vi "CRYImp wiz p2 basic format.vi"(5 "Iteration":i32, 6 "x-y settings array":T1 {"yp db ref" format="%.2f"; "ym db ref" format="%.2f"; "x db ref" format="%.2f"}, 7 "Flat data in (optional)":string, 8 "error in (no error)":errorcluster, 10 "Main info cluster":T2, 11 "Page flags":T3) -> (0 "error out":errorcluster, 1 "Data out":string[][](array[string]), 2 "Main info cluster out":T2, 3 "Page flags out":T3, 4 "x-y settings array out":T1 {"yp db ref" format="%.2f"; "ym db ref" format="%.2f"; "x db ref" format="%.2f"})   [LabVIEW 2013]
uses:
  Control/CRYImp wiz page flags.ctl
  Control/CRYImp wiz main info.ctl
  Control/CRYx-y settings array.ctl
panel:
  out "Operand_A1":bool
  in  "column width:":i32=10 caption="列宽度:"
  in  "col oth delim":string="   " caption="其他:"
  in  "column delimiter:":u16(ring) caption="aa" items=["tab", "comma", "space", "other"]
  in  "prev":bool
  in  "next":bool
  in  "cancel":bool
  in  "finish":bool
  in  "rows/cols":i32(slide) caption="aa"
  in  "file format":i32(slide)
  in  "offset cols":i32 caption="aa" min=0
  in  "offset rows":i32 caption="aa" min=0
  out "File viewer (after offset):":string[][](table) caption="aa"
  in  "cont":bool
  in  "header col":i32=1 caption="行/列:" min=1
  in  "header":bool caption="aaa"
  in  "load":bool
  in  "cntls update":bool
  in  "std hdr":bool caption="标准头包含轴"
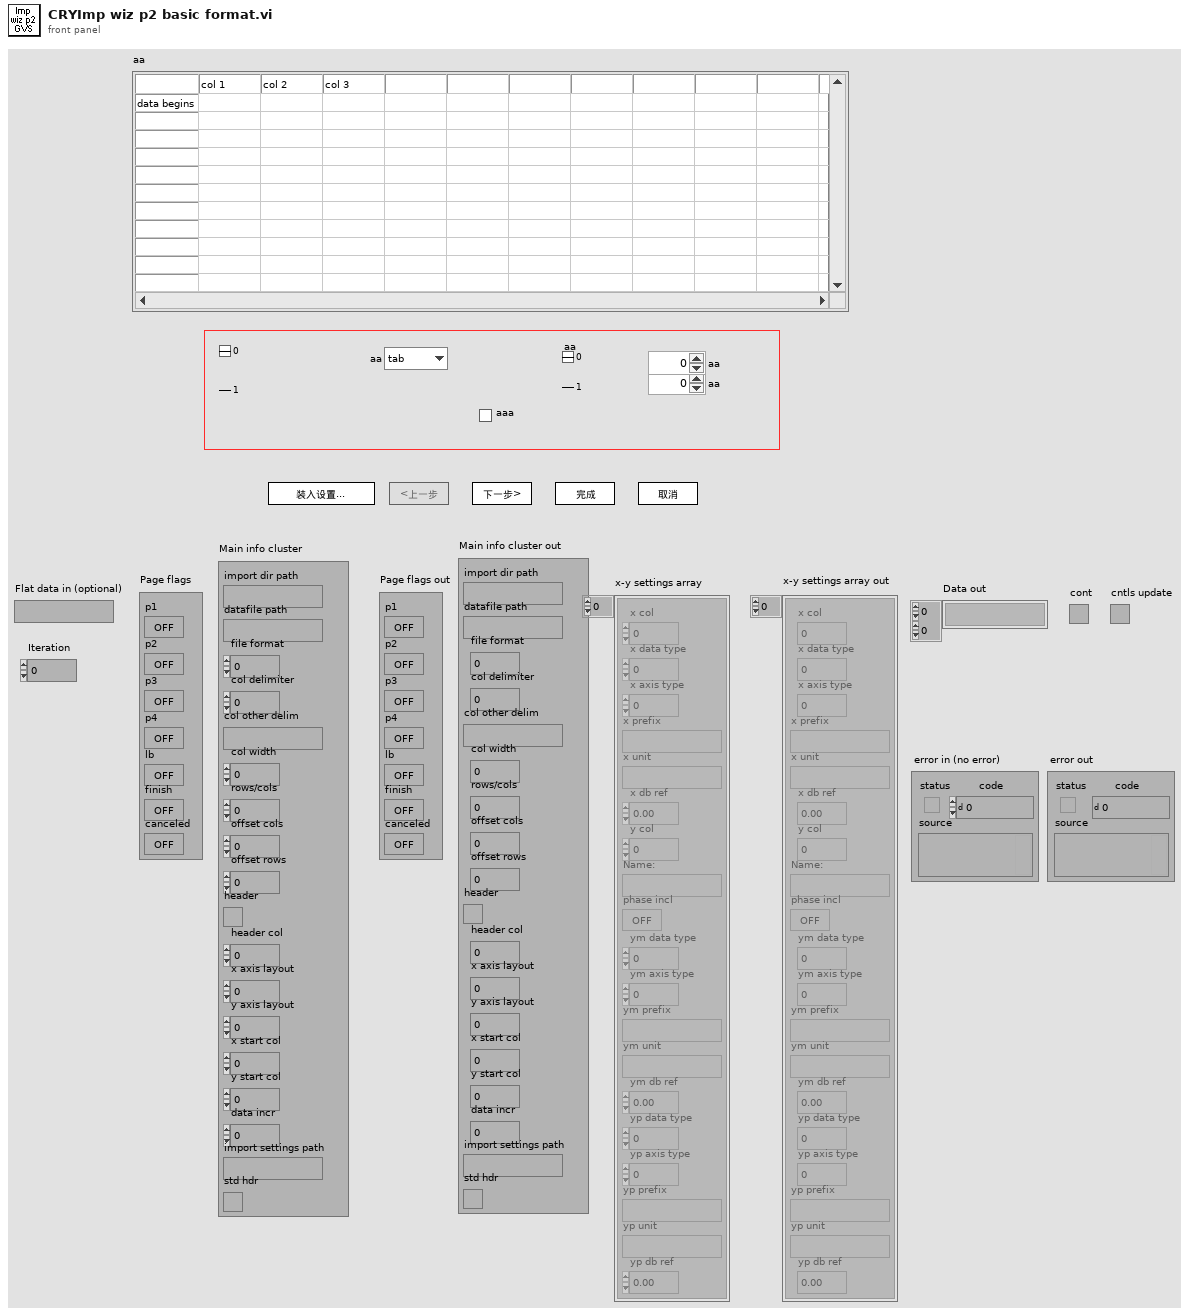
[diagram p1: front panel]
types:
  T1 = typedef "CRYx-y settings array.ctl" = cluster{"x col":i32, "x data type":u16, "x axis type":u16, "x prefix":string, "x unit":string, "x db ref":dbl, "y col":i32, "Name:":string, "phase incl":bool, "ym data type":u16, "ym axis type":u16, "ym prefix":string, "ym unit":string, "ym db ref":dbl, "yp data type":u16, "yp axis type":u16, "yp prefix":string, "yp unit":string, "yp db ref":dbl}[]
  T2 = typedef "CRYImp wiz main info.ctl" = cluster{"import dir path":path, "datafile path":path, "file format":i32, "col delimiter":i32, "col other delim":string, "col width":i32, "rows/cols":i32, "offset cols":i32, "offset rows":i32, "header":bool, "header col":i32, "x axis layout":i32, "y axis layout":i32, "x start col":i32, "y start col":i32, "data incr":i32, "import settings path":path, "std hdr":bool}
  T3 = typedef "CRYImp wiz page flags.ctl" = cluster{"p1":bool, "p2":bool, "p3":bool, "p4":bool, "lb":bool, "finish":bool, "canceled":bool}
  T4 = enum16{"read/write", "read-only", "write-only", "write-only (truncate)"}
  T5 = cluster{"file format":i32, "column delimiter:":u16, "col oth delim":string, "column width:":i32, "rows/cols":i32, "offset cols":i32, "offset rows":i32, "header":bool, "header col":i32, "std hdr":bool}
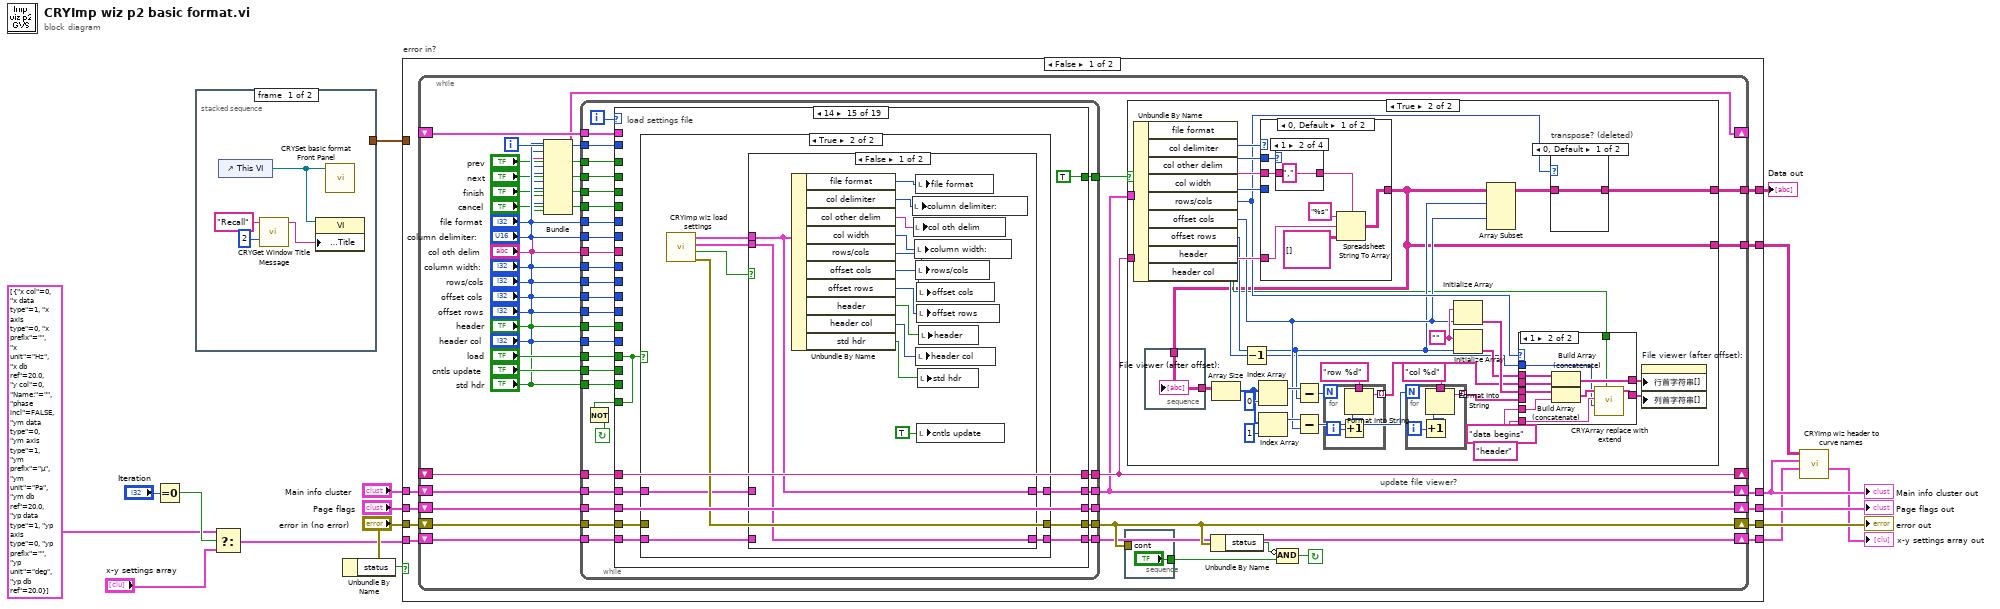
[diagram p0: block diagram]
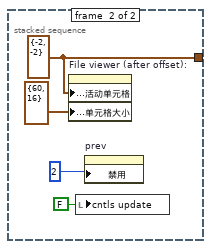
[diagram p2: hidden frame]
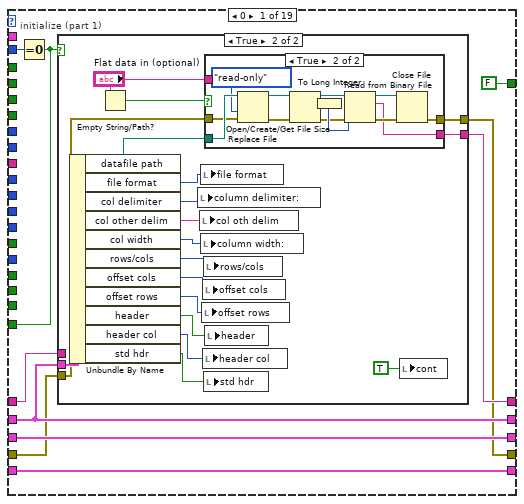
[diagram p3: hidden frame]
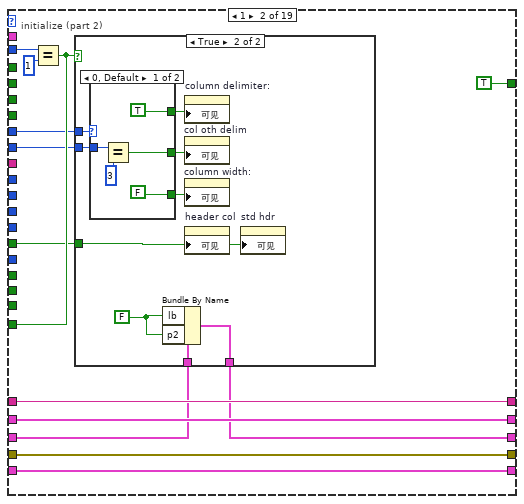
[diagram p6: hidden frame]
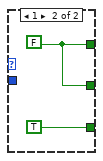
[diagram p8: hidden frame]
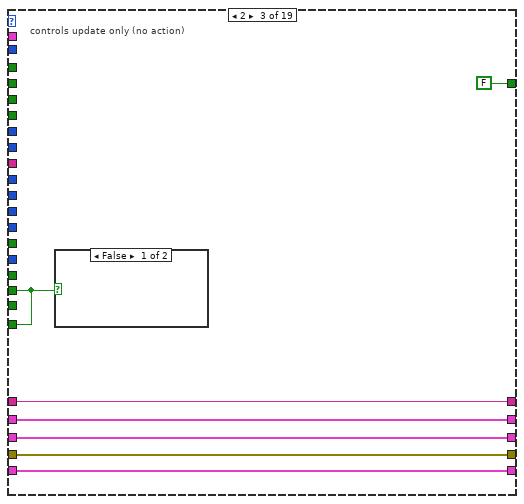
[diagram p9: hidden frame]
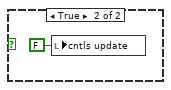
[diagram p10: hidden frame]
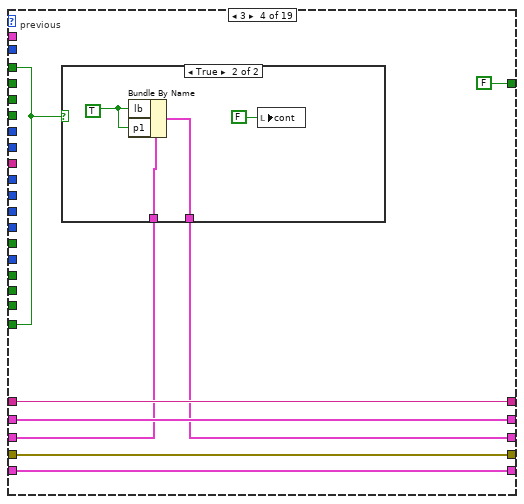
[diagram p11: hidden frame]
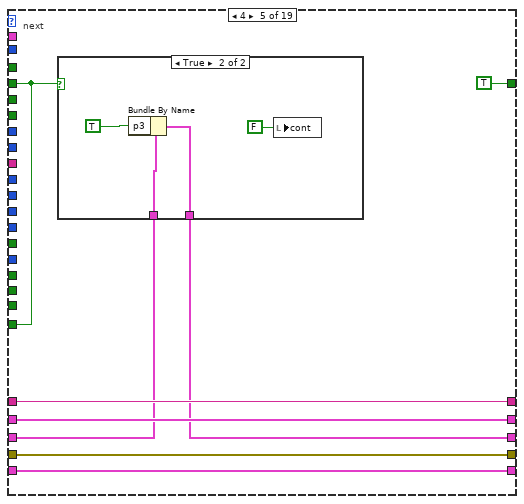
[diagram p13: hidden frame]
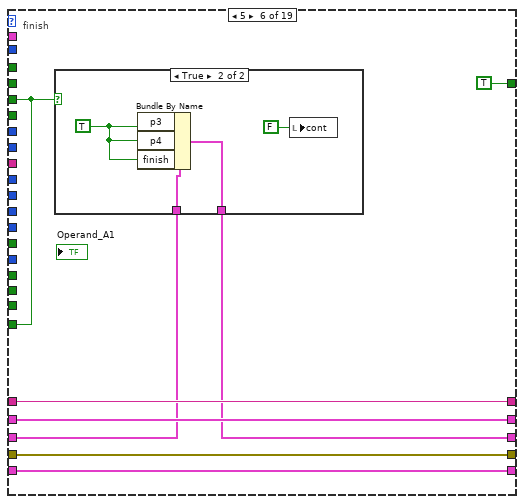
[diagram p15: hidden frame]
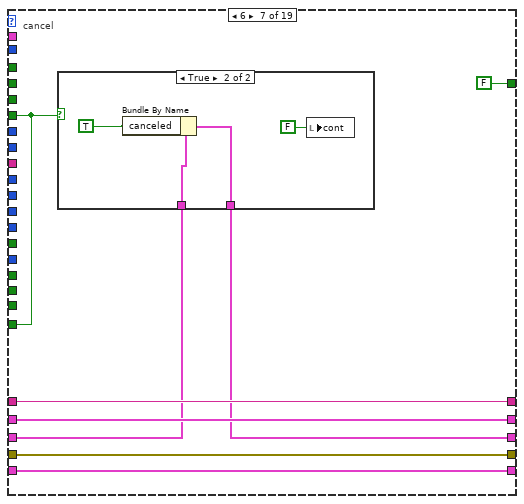
[diagram p17: hidden frame]
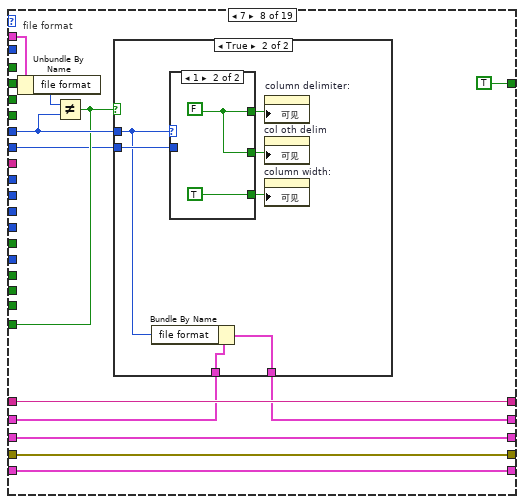
[diagram p19: hidden frame]
diagram:
  n1 = Equal To 0?(x="Iteration") -> (x = 0?=w4:bool)
  n2 = stacked-sequence {
    tunnel: [_ w24] -> w10
    frame #0 {
      n3 = control-ref of="This VI"() -> (w19:refnum<vi>)
      n4 = call "CRYGet Window Title Message.vi"("No"=2, "Kind"="Recall") -> ("Multibyte String"=w18:string)  [unwired: 4 in, 5 out]
      n5 = property class="VI"(reference=w19, "Front Panel.Title"=w18) -> ()  [unwired: 1 in, 2 out]
      n6 = call "CRYSet basic format Front Panel.vi"("Vi Ref"=w19) -> ()  [unwired: 11 in]
    }
    frame #1 {
      w24 = cluster{i32, i32} {-2, -2} ("Write Attribute")
      n7 = property on="File viewer (after offset):" class="Tbl (strict)"("活动单元格:活动单元格"=w24, "活动单元格:单元格大小"=cluster{"Width":u32, "Height":u32} {"Width"=60, "Height"=16} ("Write Attribute")) -> ()  [unwired: 2 in, 2 out]
      n8 = local write "cntls update"(FALSE ("cntls update")) -> ()
      n9 = property on="prev" class="Bool"("禁用"=u8 2 ("Write Attribute")) -> ()  [unwired: 2 in, 2 out]
    }
  }
  n10 = Select(t=T1 [{"x col"=0, "x data type"=1, "x axis type"=0, "x prefix"="", "x unit"="Hz", "x db ref"=20.0, "y col"=0, "Name:"="", "phase incl"=FALSE, "ym data type"=0, "ym axis type"=1, "ym prefix"="µ", "ym unit"="Pa", "ym db ref"=20.0, "yp data type"=1, "yp axis type"=0, "yp prefix"="", "yp unit"="deg", "yp db ref"=20.0}] ("x-y settings array"), s=w4, f="x-y settings array") -> (s? t:f=w1:T1)
  n11 = Unbundle By Name("error in (no error)") -> ("status"=w13:bool)
  n12 = case "error in?" shown="False" w13 {
    tunnel: "Main info cluster" -> [w35 w573]
    tunnel: [w32 w573] -> w8
    tunnel: "Page flags" -> [w34 w574]
    tunnel: [w31 w574] -> w15
    tunnel: "error in (no error)" -> [w33 w575]
    tunnel: [w30 w575] -> w12
    tunnel: [w29 w571] -> w11
    tunnel: w10 -> [_ _]
    tunnel: w1 -> [w28 w572]
    tunnel: [w27 w572] -> w7
    tunnel: [w26 w571] -> w9
    frame False {
      n13 = while {
        tunnel: [w37] -> w26
        shift-left: w28 -> [w39]
        shift-right: [w40] -> w27
        tunnel: [w44] -> w29
        shift-left: _ -> [w52]
        shift-right: [w51] -> _
        shift-left: _ -> [w70]
        shift-right: [w49] -> _
        shift-left: w33 -> [w54]
        shift-right: [w46] -> w30
        shift-left: w34 -> [w55]
        shift-right: [w53] -> w31
        shift-left: w35 -> [w56]
        shift-right: [w50] -> w32
        i -> [w69]
        stop <- w45 continue-if-true
        n14 = Bundle("file format"="file format", "column delimiter:"="column delimiter:", "col oth delim"="col oth delim", "column width:"="column width:", "rows/cols"="rows/cols", "offset cols"="offset cols", "offset rows"="offset rows", "header"="header", "header col"="header col", "std hdr"="std hdr") -> (w49:T5)  [unwired: 1 out]
        n15 = while {
          tunnel: "std hdr" -> [w71]
          tunnel: "cntls update" -> [w72]
          tunnel: w39 -> [w73]
          tunnel: [w74] -> w40
          tunnel: "load" -> [w75]
          tunnel: "header col" -> [w76]
          tunnel: "header" -> [w77]
          tunnel: w52 -> [w78]
          tunnel: [w79] -> w51
          tunnel: [w80] -> w46
          tunnel: w54 -> [w81]
          tunnel: [w82] -> w53
          tunnel: w55 -> [w83]
          tunnel: [w84] -> w50
          tunnel: w56 -> [w85]
          tunnel: [w86] -> w57
          tunnel: "cancel" -> [w89]
          tunnel: "finish" -> [w90]
          tunnel: "next" -> [w91]
          tunnel: "prev" -> [w92]
          tunnel: "offset rows" -> [w93]
          tunnel: "offset cols" -> [w94]
          tunnel: "rows/cols" -> [w95]
          tunnel: "column width:" -> [w96]
          tunnel: "col oth delim" -> [w97]
          tunnel: "column delimiter:" -> [w98]
          tunnel: "file format" -> [w99]
          tunnel: w69 -> [w100]
          tunnel: w70 -> [w101]
          i -> [w102]
          stop <- w88 continue-if-true
          n16 = case shown="14" w102 {
            tunnel: w101 -> [_ _ _ _ _ _ _ w245 w271 w288 w299 w310 w321 w332 _ w386 w425 w453 _]
            tunnel: w100 -> [w112 w160 _ _ _ _ _ _ _ _ _ _ _ _ _ _ _ _ _]
            tunnel: w99 -> [_ w151 _ _ _ _ _ w243 _ _ _ _ _ _ _ _ _ _ _]
            tunnel: w98 -> [_ w150 _ _ _ _ _ w239 w267 _ _ _ _ _ _ _ _ _ _]
            tunnel: w97 -> [_ _ _ _ _ _ _ _ _ w283 _ _ _ _ _ _ _ _ _]
            tunnel: w96 -> [_ _ _ _ _ _ _ _ _ _ w294 _ _ _ _ _ _ _ _]
            tunnel: w95 -> [_ _ _ _ _ _ _ _ _ _ _ w305 _ _ _ w376 _ w443 _]
            tunnel: w94 -> [_ _ _ _ _ _ _ _ _ _ _ _ w316 _ _ w375 _ w442 _]
            tunnel: w93 -> [_ _ _ _ _ _ _ _ _ _ _ _ _ w327 _ w374 _ w441 _]
            tunnel: w92 -> [_ _ _ w187 _ _ _ _ _ _ _ _ _ _ _ _ _ _ _]
            tunnel: w91 -> [_ _ _ _ w200 _ _ _ _ _ _ _ _ _ _ _ _ _ _]
            tunnel: w90 -> [_ _ _ _ _ w213 _ _ _ _ _ _ _ _ _ _ _ _ _]
            tunnel: w89 -> [_ _ _ _ _ _ w226 _ _ _ _ _ _ _ _ _ _ _ _]
            tunnel: [w111 w152 w178 w187 w200 w213 w226 w240 w266 w286 w297 w308 w319 w330 w344 w384 w423 w444 TRUE] -> w87
            tunnel: [FALSE TRUE FALSE FALSE TRUE TRUE FALSE TRUE TRUE TRUE TRUE TRUE TRUE TRUE TRUE TRUE TRUE TRUE FALSE] -> w86
            tunnel: w85 -> [w108 w158 w182 w193 w206 w219 w232 w242 w269 w285 w296 w307 w318 w329 w342 w379 w418 w450 w485]
            tunnel: [w108 w158 w182 w193 w206 w219 w232 w241 w268 w284 w295 w306 w317 w328 w341 w378 w417 w449 w485] -> w84
            tunnel: w83 -> [w109 w154 w181 w189 w202 w215 w228 w246 w272 w289 w300 w311 w322 w333 w346 w381 w422 w447 w484]
            tunnel: [w109 w153 w181 w188 w201 w214 w227 w246 w272 w289 w300 w311 w322 w333 w346 w381 w422 w447 w484] -> w82
            tunnel: w81 -> [w104 w157 w180 w190 w203 w216 w229 w247 w273 w290 w301 w312 w323 w334 w340 w380 w421 w446 w483]
            tunnel: [w105 w157 w180 w190 w203 w216 w229 w247 w273 w290 w301 w312 w323 w334 w339 w380 w421 w446 w483] -> w80
            tunnel: [w107 w155 w183 w191 w204 w217 w230 w248 w274 w291 w302 w313 w324 w335 w345 w382 w416 w448 w486] -> w79
            tunnel: w78 -> [w106 w155 w183 w191 w204 w217 w230 w248 w274 w291 w302 w313 w324 w335 w345 w382 w416 w448 w486]
            tunnel: w77 -> [_ w148 _ _ _ _ _ _ _ _ _ _ _ _ _ w383 _ _ _]
            tunnel: w76 -> [_ _ _ _ _ _ _ _ _ _ _ _ _ _ _ w373 _ w451 _]
            tunnel: w75 -> [_ _ _ _ _ _ _ _ _ _ _ _ _ _ w344 _ _ _ _]
            tunnel: [w103 w149 w179 w186 w199 w212 w225 w238 w265 w282 w293 w304 w315 w326 w338 w377 w420 w445 w482] -> w74
            tunnel: w73 -> [w103 w149 w179 w186 w199 w212 w225 w238 w265 w282 w293 w304 w315 w326 w337 w377 w420 w445 w482]
            tunnel: w72 -> [_ _ w178 _ _ _ _ _ _ _ _ _ _ _ _ _ _ _ _]
            tunnel: w71 -> [_ _ _ _ _ _ _ _ _ _ _ _ _ _ _ _ w419 _ _]
            frame 0 {
              # "initialize (part 1)"
              n17 = Equal To 0?(x=w112) -> (x = 0?=w111:bool)
              n18 = case shown="True" w111 {
                tunnel: w108 -> [_ w125]
                tunnel: [w114 w121] -> w107
                tunnel: w106 -> [w114 _]
                tunnel: [w113 w122] -> w105
                tunnel: w104 -> [w113 w118]
                frame False {
                }
                frame True {
                  n19 = Unbundle By Name(w125) -> ("datafile path"=w124:path, "file format"=w128:i32, "col delimiter"=w127:i32, "col other delim"=w126:string, "col width"=w132:i32, "rows/cols"=w131:i32, "offset cols"=w130:i32, "offset rows"=w129:i32, "header"=w120:bool, "header col"=w119:i32, "std hdr"=w115:bool)
                  n20 = Empty String/Path?(string/path="Flat data in (optional)") -> (empty?=w117:bool)
                  n21 = local write "column delimiter:"(w127) -> ()
                  n22 = local write "col oth delim"(w126) -> ()
                  n23 = local write "file format"(w128) -> ()
                  n24 = local write "column width:"(w132) -> ()
                  n25 = local write "offset rows"(w129) -> ()
                  n26 = local write "offset cols"(w130) -> ()
                  n27 = local write "header col"(w119) -> ()
                  n28 = local write "rows/cols"(w131) -> ()
                  n29 = local write "std hdr"(w115) -> ()
                  n30 = case shown="True" w117 {
                    tunnel: w124 -> [_ w146]
                    tunnel: [w134 w138] -> w122
                    tunnel: [w133 w137] -> w121
                    tunnel: w118 -> [w134 w136]
                    tunnel: "Flat data in (optional)" -> [w133 _]
                    frame False {
                    }
                    frame True {
                      n31 = Open/Create/Replace File(file path (use dialog)=w146, error in=w136, access (0:read/write)=T4."read-only" ("open mode (0)")) -> (refnum out=w144:refnum<file>, error out=w147:errorcluster)  [unwired: 4 out]
                      n32 = Get File Size(file=w144, error in=w147) -> (refnum out=w141:refnum<file>, size (in bytes)=w135:i64, 0:w142:errorcluster)
                      n33 = To Long Integer(number=w135) -> (32bit integer=w143:i32)
                      n34 = Read from Binary File(8:w142, 10:w143, 11:w141) -> (0:w139:errorcluster, 2:w137:string, 3:w140:refnum<file>)  [unwired: 4 out]
                      n35 = Close File(refnum=w140, error in=w139) -> (error out=w138:errorcluster)  [unwired: 1 out]
                    }
                  }
                  n36 = local write "header"(w120) -> ()
                  n37 = local write "cont"(TRUE ("cont")) -> ()
                }
              }
            }
            frame 1 {
              # "initialize (part 2)"
              n38 = Equal?(x=w160, y=1) -> (x = y?=w152:bool)
              n39 = case shown="True" w152 {
                tunnel: w154 -> [w161 w169]
                tunnel: [w161 w168] -> w153
                tunnel: w151 -> [_ w167]
                tunnel: w150 -> [_ w166]
                tunnel: w148 -> [_ w162]
                frame False {
                }
                frame True {
                  w170 = FALSE ("Bundle Element")
                  n40 = case shown="0, Default" w167 {
                    tunnel: w166 -> [w175 _]
                    tunnel: [w173 w177] -> w165
                    tunnel: [TRUE ("Bundle Element") w177] -> w164
                    tunnel: [FALSE ("Bundle Element") TRUE ("Bundle Element")] -> w163
                    frame 0, Default {
                      n41 = Equal?(x=w175, y=3 ("column delimiter:")) -> (x = y?=w173:bool)
                    }
                    frame 1 {
                      w177 = FALSE ("Bundle Element")
                    }
                  }
                  n42 = Bundle By Name(cluster=w169, "lb"=w170, "p2"=w170) -> (w168:T3)
                  n43 = property on="column delimiter:" class="Ring (strict)"("可见"=w164) -> ()  [unwired: 2 in, 2 out]
                  n44 = property on="col oth delim" class="Str"("可见"=w165) -> ()  [unwired: 2 in, 2 out]
                  n45 = property on="column width:" class="DigNum (strict)"("可见"=w163) -> ()  [unwired: 2 in, 2 out]
                  n46 = property on="header col" class="DigNum (strict)"("可见"=w162) -> ()  [unwired: 2 in, 2 out]
                  n47 = property on="std hdr" class="Bool (strict)"("可见"=w162) -> ()  [unwired: 2 in, 2 out]
                }
              }
            }
            frame 2 {
              # "controls update only (no action)"
              n48 = case shown="False" w178 {
                frame False {
                }
                frame True {
                  n49 = local write "cntls update"(FALSE ("cntls update")) -> ()
                }
              }
            }
            frame 3 {
              # "previous"
              n50 = case shown="True" w187 {
                tunnel: w189 -> [w194 w197]
                tunnel: [w194 w196] -> w188
                frame False {
                }
                frame True {
                  w198 = TRUE ("Bundle Element")
                  n51 = Bundle By Name(cluster=w197, "lb"=w198, "p1"=w198) -> (w196:T3)
                  n52 = local write "cont"(FALSE ("cont")) -> ()
                }
              }
            }
            frame 4 {
              # "next"
              n53 = case shown="True" w200 {
                tunnel: w202 -> [w207 w211]
                tunnel: [w207 w210] -> w201
                frame False {
                }
                frame True {
                  n54 = Bundle By Name(cluster=w211, "p3"=TRUE ("Bundle Element")) -> (w210:T3)
                  n55 = local write "cont"(FALSE ("cont")) -> ()
                }
              }
            }
            frame 5 {
              # "finish"
              n56 = case shown="True" w213 {
                tunnel: w215 -> [w220 w224]
                tunnel: [w220 w223] -> w214
                frame False {
                }
                frame True {
                  w222 = TRUE ("Bundle Element")
                  n57 = Bundle By Name(cluster=w224, "p3"=w222, "p4"=w222, "finish"=w222) -> (w223:T3)
                  n58 = local write "cont"(FALSE ("cont")) -> ()
                }
              }
            }
            frame 6 {
              # "cancel"
              n59 = case shown="True" w226 {
                tunnel: w228 -> [w233 w237]
                tunnel: [w233 w236] -> w227
                frame False {
                }
                frame True {
                  n60 = Bundle By Name(cluster=w237, "canceled"=TRUE ("Bundle Element")) -> (w236:T3)
                  n61 = local write "cont"(FALSE ("cont")) -> ()
                }
              }
            }
            frame 7 {
              # "file format"
              n62 = Unbundle By Name(w245) -> ("file format"=w244:i32)
              n63 = Not Equal?(x=w244, y=w243) -> (x != y?=w240:bool)
              n64 = case shown="True" w240 {
                tunnel: w243 -> [_ w251]
                tunnel: w242 -> [w250 w257]
                tunnel: [w250 w256] -> w241
                tunnel: w239 -> [_ w252]
                frame False {
                }
                frame True {
                  n65 = Bundle By Name(cluster=w257, "file format"=w251) -> (w256:T2)
                  n66 = case shown="1" w251 {
                    tunnel: w252 -> [w262 _]
                    tunnel: [w260 w264] -> w255
                    tunnel: [TRUE ("Bundle Element") w264] -> w254
                    tunnel: [FALSE ("Bundle Element") TRUE ("Bundle Element")] -> w253
                    frame 0, Default {
                      n67 = Equal?(x=w262, y=3 ("column delimiter:")) -> (x = y?=w260:bool)
                    }
                    frame 1 {
                      w264 = FALSE ("Bundle Element")
                    }
                  }
                  n68 = property on="column delimiter:" class="Ring (strict)"("可见"=w254) -> ()  [unwired: 2 in, 2 out]
                  n69 = property on="col oth delim" class="Str"("可见"=w255) -> ()  [unwired: 2 in, 2 out]
                  n70 = property on="column width:" class="DigNum (strict)"("可见"=w253) -> ()  [unwired: 2 in, 2 out]
                }
              }
            }
            frame 8 {
              # "column delimitter"
              n71 = Unbundle By Name(w271) -> ("column delimiter:"=w270:u16)
              n72 = Not Equal?(x=w270, y=w267) -> (x != y?=w266:bool)
              n73 = case shown="True" w266 {
                tunnel: w269 -> [w276 w281]
                tunnel: [w276 w280] -> w268
                tunnel: w267 -> [_ w278]
                frame False {
                }
                frame True {
                  n74 = Bundle By Name(cluster=w281, "col delimiter"=w278) -> (w280:T2)
                  n75 = Equal?(x=w278, y=3 ("column delimiter:")) -> (x = y?=w277:bool)
                  n76 = property on="col oth delim" class="Str"("可见"=w277) -> ()  [unwired: 2 in, 2 out]
                }
              }
            }
            frame 9 {
              # "column other delimitter"
              n77 = Unbundle By Name(w288) -> ("col oth delim"=w287:string)
              n78 = Not Equal?(x=w287, y=w283) -> (x != y?=w286:bool)
              n79 = Bundle By Name(cluster=w285, "col other delim"=w283) -> (w284:T2)
            }
            frame 10 {
              # "column width"
              n80 = Unbundle By Name(w299) -> ("column width:"=w298:i32)
              n81 = Not Equal?(x=w298, y=w294) -> (x != y?=w297:bool)
              n82 = Bundle By Name(cluster=w296, "col width"=w294) -> (w295:T2)
            }
            frame 11 {
              # "rows/cols"
              n83 = Unbundle By Name(w310) -> ("rows/cols"=w309:i32)
              n84 = Not Equal?(x=w309, y=w305) -> (x != y?=w308:bool)
              n85 = Bundle By Name(cluster=w307, "rows/cols"=w305) -> (w306:T2)
            }
            frame 12 {
              # "offset columns"
              n86 = Unbundle By Name(w321) -> ("offset cols"=w320:i32)
              n87 = Not Equal?(x=w320, y=w316) -> (x != y?=w319:bool)
              n88 = Bundle By Name(cluster=w318, "offset cols"=w316) -> (w317:T2)
            }
            frame 13 {
              # "offset rows"
              n89 = Unbundle By Name(w332) -> ("offset rows"=w331:i32)
              n90 = Not Equal?(x=w331, y=w327) -> (x != y?=w330:bool)
              n91 = Bundle By Name(cluster=w329, "offset rows"=w327) -> (w328:T2)
            }
            frame 14 {
              # "load settings file"
              n92 = case shown="True" w344 {
                tunnel: [w349 w354] -> w341
                tunnel: w342 -> [w349 w353]
                tunnel: [w348 w356] -> w339
                tunnel: w340 -> [w348 _]
                tunnel: [w347 w351] -> w338
                tunnel: w337 -> [w347 w350]
                frame False {
                }
                frame True {
                  n93 = call "CRYImp wiz load settings.vi"() -> ("error out"=w356:errorcluster, "Canceled"=w357:bool, "x-y settings array out"=w352:T1, "Main info cluster out"=w355:T2)  [unwired: 8 in]
                  n94 = case shown="False" w357 {
                    tunnel: w355 -> [w361 _]
                    tunnel: [w361 w372] -> w354
                    tunnel: w353 -> [_ w372]
                    tunnel: w352 -> [w360 _]
                    tunnel: [w360 w371] -> w351
                    tunnel: w350 -> [_ w371]
                    frame False {
                      n95 = Unbundle By Name(w361) -> ("file format"=w366:i32, "col delimiter"=w365:i32, "col other delim"=w364:string, "col width"=w370:i32, "rows/cols"=w369:i32, "offset cols"=w368:i32, "offset rows"=w367:i32, "header"=w363:bool, "header col"=w362:i32, "std hdr"=w358:bool)
                      n96 = local write "column delimiter:"(w365) -> ()
                      n97 = local write "col oth delim"(w364) -> ()
                      n98 = local write "column width:"(w370) -> ()
                      n99 = local write "file format"(w366) -> ()
                      n100 = local write "rows/cols"(w369) -> ()
                      n101 = local write "header col"(w362) -> ()
                      n102 = local write "offset cols"(w368) -> ()
                      n103 = local write "offset rows"(w367) -> ()
                      n104 = local write "cntls update"(TRUE ("cntls update")) -> ()
                      n105 = local write "std hdr"(w358) -> ()
                      n106 = local write "header"(w363) -> ()
                    }
                    frame True {
                    }
                  }
                }
              }
            }
            frame 15 {
              # "include header"
              n107 = Unbundle By Name(w386) -> ("header"=w385:bool)
              n108 = Exclusive Or(1:w383, 2:w385) -> (0:w384:bool)
              n109 = case shown="True" w384 {
                tunnel: w383 -> [_ w395]
                tunnel: w379 -> [w388 w397]
                tunnel: [w388 w396] -> w378
                tunnel: w376 -> [_ w394]
                tunnel: w375 -> [_ w392]
                tunnel: w374 -> [_ w393]
                tunnel: w373 -> [_ w389]
                frame False {
                }
                frame True {
                  n110 = case shown="0, Default" w394 {
                    tunnel: w393 -> [w401 w408]
                    tunnel: w392 -> [w399 w410]
                    tunnel: w389 -> [w403 w412]
                    tunnel: [w400 w408] -> w390
                    tunnel: [w399 w409] -> w391
                    frame 0, Default {
                      n111 = Decrement(x=w403) -> (x-1=w398:i32)
                      n112 = Equal?(x=w401, y=w398) -> (x = y?=w402:bool)
                      n113 = case shown="True" w402 {
                        tunnel: w401 -> [w404 w406]
                        tunnel: [w404 w405] -> w400
                        frame False {
                        }
                        frame True {
                          n114 = Increment(x=w406) -> (x+1=w405:i32)
                        }
                      }
                    }
                    frame 1 {
                      n115 = Decrement(x=w412) -> (x-1=w407:i32)
                      n116 = Equal?(x=w410, y=w407) -> (x = y?=w411:bool)
                      n117 = case shown="False" w411 {
                        tunnel: w410 -> [w413 w415]
                        tunnel: [w413 w414] -> w409
                        frame False {
                        }
                        frame True {
                          n118 = Increment(x=w415) -> (x+1=w414:i32)
                        }
                      }
                    }
                  }
                  n119 = local write "offset rows"(w390) -> ()
                  n120 = local write "offset cols"(w391) -> ()
                  n121 = Bundle By Name(cluster=w397, "header"=w395, "offset cols"=w391, "offset rows"=w390, "header col"=w389) -> (w396:T2)
                  n122 = property on="header col" class="DigNum (strict)"("可见"=w395) -> ()  [unwired: 2 in, 2 out]
                  n123 = property on="std hdr" class="Bool (strict)"("可见"=w395) -> ()  [unwired: 2 in, 2 out]
                }
              }
            }
            frame 16 {
              # "standard header"
              n124 = Unbundle By Name(w425) -> ("std hdr"=w424:bool)
              n125 = Exclusive Or(1:w419, 2:w424) -> (0:w423:bool)
              n126 = case shown="True" w423 {
                tunnel: w419 -> [_ w431]
                tunnel: w418 -> [w427 w430]
                tunnel: [w427 w429] -> w417
                tunnel: w416 -> [_ w428]
                frame False {
                }
                frame True {
                  n127 = case shown="True" w431 {
                    tunnel: w430 -> [w434 w439]
                    tunnel: [w433 w435] -> w429
                    tunnel: w428 -> [_ w440]
                    frame False {
                      n128 = Bundle By Name(cluster=w434, "std hdr"=FALSE ("Bundle Element")) -> (w433:T2)
                    }
                    frame True {
                      n129 = call "CRYStd header find.vi"("Flat data"=w440, "Main info cluster"=w439) -> ("Main info cluster out"=w435:T2)  [unwired: 9 in]
                      n130 = Unbundle By Name(w435) -> ("offset cols"=w437:i32, "offset rows"=w438:i32, "header col"=w436:i32)
                      n131 = local write "offset rows"(w438) -> ()
                      n132 = local write "offset cols"(w437) -> ()
                      n133 = local write "header col"(w436) -> ()
                    }
                  }
                }
              }
            }
            frame 17 {
              # "header column"
              n134 = Unbundle By Name(w453) -> ("header col"=w452:i32)
              n135 = Not Equal?(x=w452, y=w451) -> (x != y?=w444:bool)
              n136 = case shown="True" w444 {
                tunnel: w451 -> [_ w458]
                tunnel: w450 -> [w455 w463]
                tunnel: [w455 w462] -> w449
                tunnel: w443 -> [_ w461]
                tunnel: w442 -> [_ w460]
                tunnel: w441 -> [_ w459]
                frame False {
                }
                frame True {
                  n137 = case shown="0, Default" w461 {
                    tunnel: w459 -> [w467 w474]
                    tunnel: w460 -> [w465 w476]
                    tunnel: w458 -> [w469 w478]
                    tunnel: [w466 w474] -> w456
                    tunnel: [w465 w475] -> w457
                    frame 0, Default {
                      n138 = Decrement(x=w469) -> (x-1=w464:i32)
                      n139 = Equal?(x=w467, y=w464) -> (x = y?=w468:bool)
                      n140 = case shown="True" w468 {
                        tunnel: w467 -> [w470 w472]
                        tunnel: [w470 w471] -> w466
                        frame False {
                        }
                        frame True {
                          n141 = Increment(x=w472) -> (x+1=w471:i32)
                        }
                      }
                    }
                    frame 1 {
                      n142 = Decrement(x=w478) -> (x-1=w473:i32)
                      n143 = Equal?(x=w476, y=w473) -> (x = y?=w477:bool)
                      n144 = case shown="True" w477 {
                        tunnel: w476 -> [w479 w481]
                        tunnel: [w479 w480] -> w475
                        frame False {
                        }
                        frame True {
                          n145 = Increment(x=w481) -> (x+1=w480:i32)
                        }
                      }
                    }
                  }
                  n146 = local write "offset rows"(w456) -> ()
                  n147 = local write "offset cols"(w457) -> ()
                  n148 = Bundle By Name(cluster=w463, "offset cols"=w457, "offset rows"=w456, "header col"=w458) -> (w462:T2)
                }
              }
            }
            frame Default {
              # "idle"
              n149 = Wait (ms)(milliseconds to wait=u32 150) -> ()  [unwired: 1 out]
            }
          }
          n150 = Not(x=w87) -> (.not. x?=w88:bool)
        }
        n151 = stacked-sequence {
          tunnel: ["cont"] -> w48
          tunnel: w46 -> [_]
          frame #0 {
          }
        }
        n152 = case "update file viewer?" shown="True" w57 {
          tunnel: w51 -> [_ w521]
          tunnel: w50 -> [_ w525]
          tunnel: [w491 w519] -> w44
          tunnel: [w491 w492] -> w37
          frame False {
            w491 = string[][] []
          }
          frame True {
            w512 = ""
            n153 = Unbundle By Name(w525) -> ("file format"=w524:i32, "col delimiter"=w523:i32, "col other delim"=w522:string, "col width"=w520:i32, "rows/cols"=w511:i32, "offset cols"=w498:i32, "offset rows"=w497:i32, "header"=w495:bool, "header col"=w494:i32)
            n154 = Decrement(x=w494) -> (x-1=w493:i32)
            n155 = case shown="0, Default" w524 {
              tunnel: w523 -> [w563 _]
              tunnel: w522 -> [w562 _]
              tunnel: w521 -> [w558 w569]
              tunnel: w520 -> [_ w570]
              tunnel: [w557 w568] -> w492
              frame 0, Default {
                n156 = case shown="1" w563 {
                  tunnel: w562 -> [_ _ _ w567]
                  tunnel: ["\t" "," " " w567] -> w559
                  frame 0, Default {
                  }
                  frame 1 {
                  }
                  frame 2 {
                  }
                  frame 3 {
                  }
                }
                n157 = Spreadsheet String To Array(delimiter (Tab)=w559, format string="%s", spreadsheet string=w558, array type (2D Dbl)=string[][] []) -> (array=w557:string[][])
              }
              frame 1 {
                n158 = call "CRYFixed column width parse.vi"("Data string"=w569, "Fixed column width"=w570) -> ("2D string array"=w568:string[][])  [unwired: 9 in]
              }
            }
            n159 = stacked-sequence {
              tunnel: w492 -> [w546]
              tunnel: [w546] -> w513
              frame #0 {
                "File viewer (after offset):" <- w546
              }
            }
            n160 = Array Size(array=w513) -> (size(s)=w514:i32[])
            n161 = Index Array(array=w514, index=0 ("Index")) -> (element=w502:i32)
            n162 = Index Array(array=w514, index=1 ("Index")) -> (element=w503:i32)
            n163 = Subtract(x=w502, y=w497) -> (x-y=w501:i32)
            n164 = Subtract(x=w503, y=w498) -> (x-y=w500:i32)
            n165 = for {
              N: w501 -> [_]
              tunnel: "row %d" -> [w552]
              tunnel: [w551] -> w505 mode=indexing
              i -> [w554]
              n166 = Increment(x=w554) -> (x+1=w553:i32)
              n167 = Format Into String(format string=w552, w553) -> (resulting string=w551:string)  [unwired: 2 in, 1 out]
            }
            n168 = for {
              N: w500 -> [_]
              tunnel: "col %d" -> [w548]
              tunnel: [w547] -> w507 mode=indexing
              i -> [w550]
              n169 = Increment(x=w550) -> (x+1=w549:i32)
              n170 = Format Into String(format string=w548, w549) -> (resulting string=w547:string)  [unwired: 2 in, 1 out]
            }
            n171 = Initialize Array(w512, w498) -> (w508:string[])
            n172 = Initialize Array(w512, w497) -> (w506:string[])
            n173 = Array Subset(array=w492, index (row)=w497, index (col)=w498) -> (w499:string[][])  [unwired: 2 in]
            n174 = case shown="1" w511 {
              tunnel: [w531 w540] -> w510
              tunnel: [w529 w543] -> w509
              tunnel: w508 -> [w535 w545]
              tunnel: w507 -> [w534 _]
              tunnel: w506 -> [w533 w544]
              tunnel: w505 -> [_ w542]
              tunnel: "data begins" -> [w532 w541]
              tunnel: "header" -> [w528 w538]
              tunnel: w495 -> [w527 w537]
              tunnel: w493 -> [w526 w536]
              frame 0, Default {
                n175 = Build Array (concatenate)(w533, w532) -> (w530:string[])
                n176 = Build Array (concatenate)(w535, w534) -> (w531:string[])
                n177 = call "CRYArray replace with extend.vi"("Enable (T)"=w527, "Index"=w526, "String element"=w528, "String array"=w530) -> ("String array out"=w529:string[])  [unwired: 7 in]
              }
              frame 1 {
                n178 = Build Array (concatenate)(w544, w542) -> (w543:string[])
                n179 = Build Array (concatenate)(w545, w541) -> (w539:string[])
                n180 = call "CRYArray replace with extend.vi"("Enable (T)"=w537, "Index"=w536, "String element"=w538, "String array"=w539) -> ("String array out"=w540:string[])  [unwired: 7 in]
              }
            }
            n181 = case "transpose? (deleted)" shown="0, Default" w511 {
              tunnel: w499 -> [w555 w556]
              tunnel: [w555 w556] -> w519
              frame 0, Default {
              }
              frame 1 {
              }
            }
            n182 = property on="File viewer (after offset):" class="Tbl (strict)"("行首字符串[]"=w509, "列首字符串[]"=w510) -> ()  [unwired: 2 in, 2 out]
          }
        }
        n183 = Unbundle By Name(w46) -> ("status"=w47:bool)
        n184 = Compound Arithmetic op=AND(invert w47, w48) -> (w45:bool)
      }
    }
    frame True {
      w571 = string[][] []
    }
  }
  "Page flags out" <- w15
  "Main info cluster out" <- w8
  "error out" <- w12
  "Data out" <- w11
  n185 = call "CRYImp wiz header to curve names.vi"("x-y settings array"=w7, "Main info cluster"=w8, "Data file table"=w9) -> ("x-y settings array out"=→"x-y settings array out":T1)  [unwired: 8 in]
